vi "编辑控件.vi"(11 "控件类型":string) -> ()   [LabVIEW 2020]
panel:
  in  "图片路径":path
  in  "修改":bool
  in  "删除":bool
  in  "增加":bool
  in  "控件列表":i32(listbox)
  out "图片预览":picture
  in  "程序文本":string
  in  "关键字":string
  in  "控件名称":string
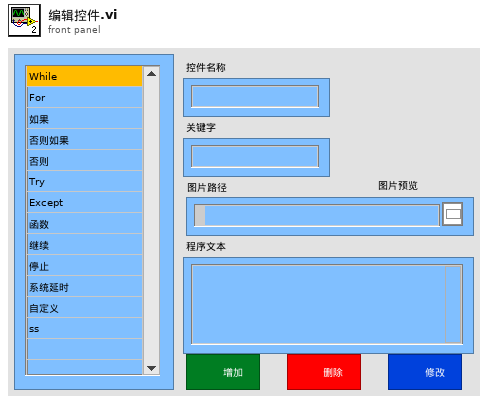
[diagram p1: front panel]
types:
  T1 = typedef "imagedata.ctl" = cluster{"image type":i32, "image depth":i32, "image":u8[], "mask":u8[], "colors":u32[], "Rectangle":cluster{"left":i16, "top":i16, "right":i16, "bottom":i16}}
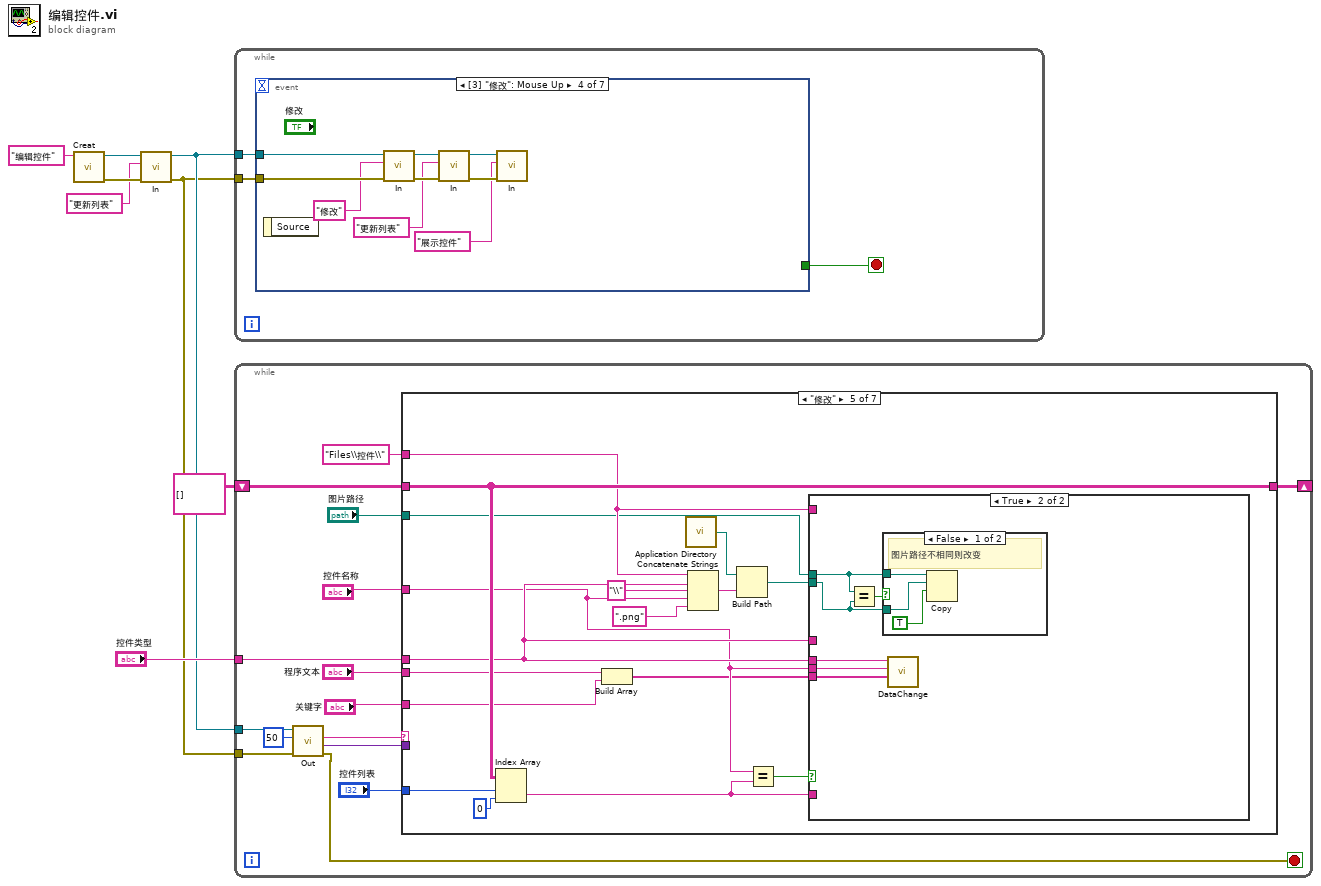
[diagram p0: block diagram]
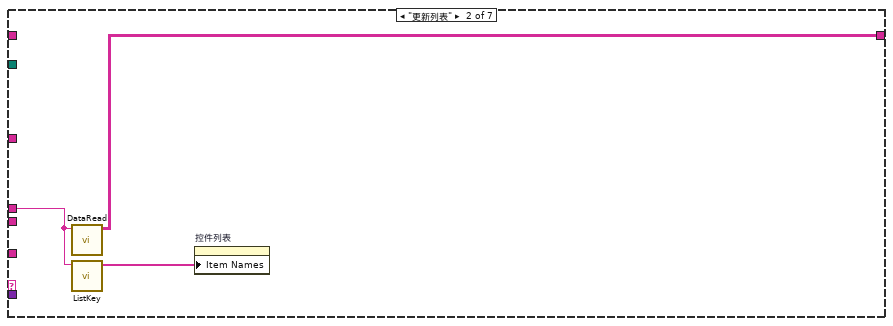
[diagram p3: hidden frame]
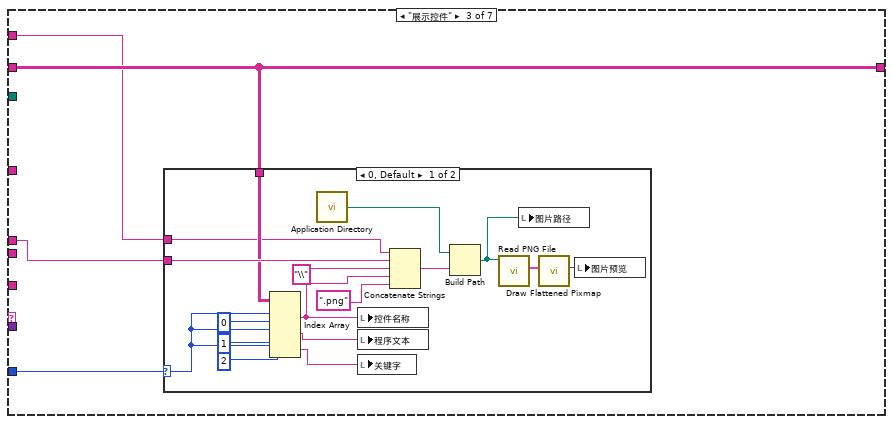
[diagram p4: hidden frame]
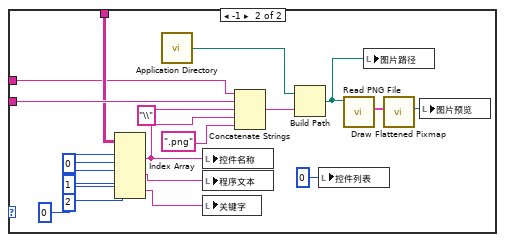
[diagram p5: hidden frame]
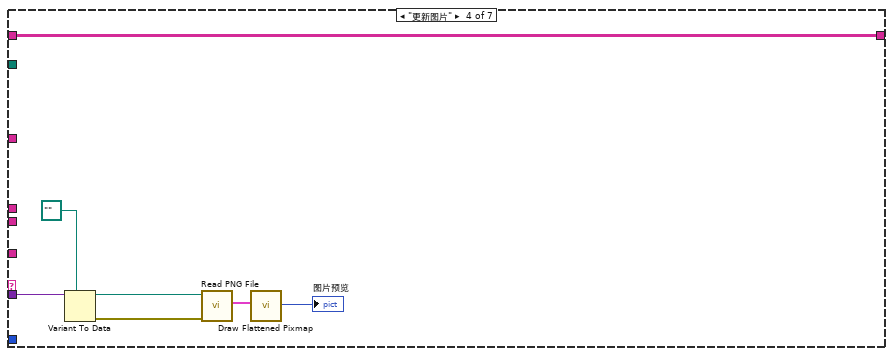
[diagram p6: hidden frame]
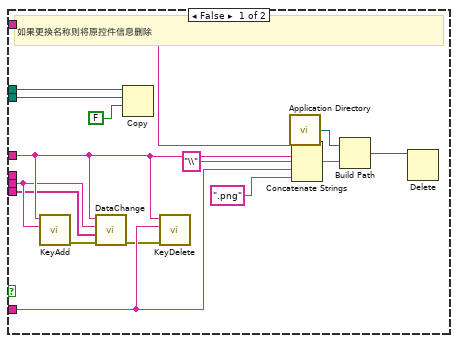
[diagram p7: hidden frame]
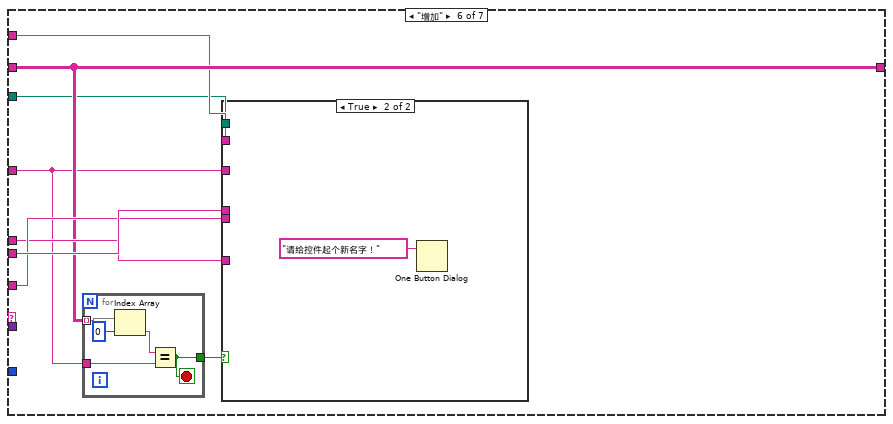
[diagram p9: hidden frame]
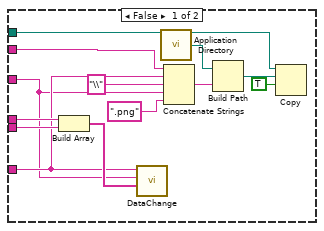
[diagram p10: hidden frame]
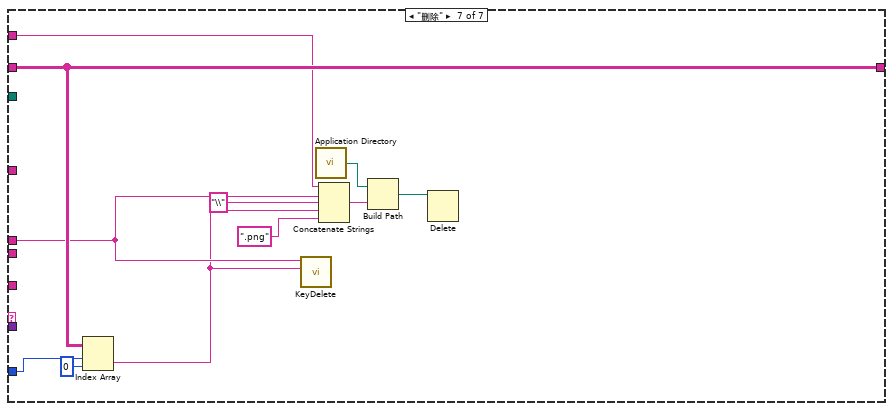
[diagram p11: hidden frame]
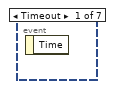
[diagram p12: hidden frame]
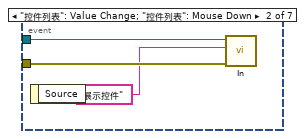
[diagram p13: hidden frame]
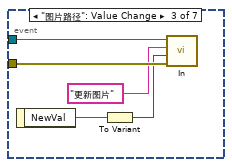
[diagram p14: hidden frame]
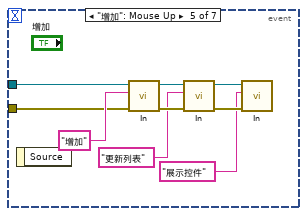
[diagram p15: hidden frame]
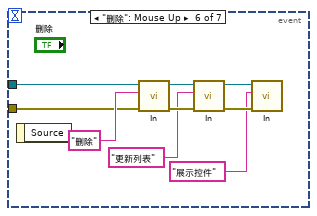
[diagram p16: hidden frame]
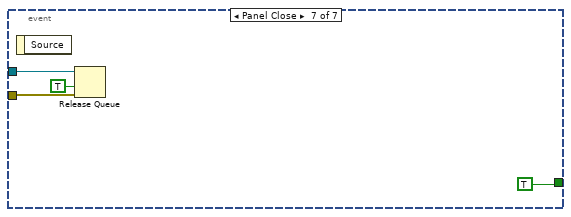
[diagram p17: hidden frame]
diagram:
  n1 = call "Creat.vi"("名称"="编辑控件") -> ("错误输出"=w2:errorcluster, "队列输出"=w5:refnum<queue>)  [unwired: 9 in]
  n2 = call "In.vi"("错误输入"=w2, "指令"="更新列表", "队列"=w5) -> ("错误输出"=w3:errorcluster, "队列输出"=w4:refnum<queue>)  [unwired: 7 in]
  n3 = while {
    tunnel: w4 -> [w11]
    tunnel: w3 -> [w10]
    stop <- w9 stop-if-true
    n4 = event shown="[3] \"修改\": Mouse Up" {
      selector: _ -> [_ _ _ _ _ _ _]
      dyn-events: _ -> [_ _ _ _ _ _ _]
      timeout: _ -> [_ _ _ _ _ _ _]
      tunnel: w11 -> [_ w14 w19 w28 w30 w39 w49]
      tunnel: w10 -> [_ w13 w18 w27 w29 w38 w48]
      tunnel: [_ _ _ _ _ _ TRUE] -> w9
      event Timeout {
        n5 = event-data() -> ()  [unwired: 1 in, 1 out]
      }
      event "控件列表": Value Change; "控件列表": Mouse Down {
        n6 = event-data() -> ()  [unwired: 1 in, 1 out]
        n7 = call "In.vi"("错误输入"=w13, "指令"="展示控件", "队列"=w14) -> ()  [unwired: 7 in, 2 out]
      }
      event "图片路径": Value Change {
        n8 = event-data() -> ("NewVal"=w17:path)  [unwired: 1 in]
        n9 = To Variant(anything=w17) -> (Variant=w15:variant)
        n10 = call "In.vi"("错误输入"=w18, "数据"=w15, "指令"="更新图片", "队列"=w19) -> ()  [unwired: 6 in, 2 out]
      }
      event "修改": Mouse Up {
        n11 = event-data() -> ()  [unwired: 1 in, 1 out]
        n12 = call "In.vi"("错误输入"=w27, "指令"="修改", "队列"=w28) -> ("错误输出"=w24:errorcluster, "队列输出"=w25:refnum<queue>)  [unwired: 7 in]
        n13 = call "In.vi"("错误输入"=w24, "指令"="更新列表", "队列"=w25) -> ("错误输出"=w22:errorcluster, "队列输出"=w23:refnum<queue>)  [unwired: 7 in]
        n14 = call "In.vi"("错误输入"=w22, "指令"="展示控件", "队列"=w23) -> ()  [unwired: 7 in, 2 out]
      }
      event "增加": Mouse Up {
        n15 = event-data() -> ()  [unwired: 1 in, 1 out]
        n16 = call "In.vi"("错误输入"=w29, "指令"="增加", "队列"=w30) -> ("错误输出"=w35:errorcluster, "队列输出"=w36:refnum<queue>)  [unwired: 7 in]
        n17 = call "In.vi"("错误输入"=w35, "指令"="更新列表", "队列"=w36) -> ("错误输出"=w33:errorcluster, "队列输出"=w34:refnum<queue>)  [unwired: 7 in]
        n18 = call "In.vi"("错误输入"=w33, "指令"="展示控件", "队列"=w34) -> ()  [unwired: 7 in, 2 out]
      }
      event "删除": Mouse Up {
        n19 = event-data() -> ()  [unwired: 1 in, 1 out]
        n20 = call "In.vi"("错误输入"=w38, "指令"="删除", "队列"=w39) -> ("错误输出"=w44:errorcluster, "队列输出"=w45:refnum<queue>)  [unwired: 7 in]
        n21 = call "In.vi"("错误输入"=w44, "指令"="更新列表", "队列"=w45) -> ("错误输出"=w42:errorcluster, "队列输出"=w43:refnum<queue>)  [unwired: 7 in]
        n22 = call "In.vi"("错误输入"=w42, "指令"="展示控件", "队列"=w43) -> ()  [unwired: 7 in, 2 out]
      }
      event Panel Close {
        n23 = event-data() -> ()  [unwired: 1 in, 1 out]
        n24 = Release Queue(queue=w49, force destroy? (F)=TRUE ("强制销毁？(F)"), error in (no error)=w48) -> ()  [unwired: 3 out]
      }
    }
  }
  n25 = while {
    tunnel: w4 -> [w58]
    tunnel: w3 -> [w57]
    shift-right: [w65] -> _
    shift-left: string[][] [] ("数据") -> [w64]
    tunnel: "控件类型" -> [w63]
    stop <- w54 stop-if-true
    n26 = call "Out.vi"("错误输入"=w57, "超时毫秒(-1)"=50, "队列"=w58) -> ("错误输出"=w54:errorcluster, "数据"=w55:variant, "指令"=w56:string)  [unwired: 5 in, 1 out]
    n27 = case shown="\"修改\"" w56 {
      tunnel: w55 -> [_ _ _ w110 _ _ _]
      tunnel: [w66 w68 w72 w114 w128 w161 w194] -> w65
      tunnel: w64 -> [w66 _ w72 w114 w128 w161 w194]
      tunnel: w63 -> [_ w69 w73 _ w118 w162 w187]
      tunnel: "控件名称" -> [_ _ _ _ w117 w160 _]
      tunnel: "程序文本" -> [_ _ _ _ w126 w164 _]
      tunnel: "关键字" -> [_ _ _ _ w125 w163 _]
      tunnel: "控件列表" -> [_ _ w71 _ w124 _ w193]
      tunnel: "Files\\控件\\" ("名称或相对路径") -> [_ _ w70 _ w121 w158 w184]
      tunnel: "图片路径" -> [_ _ _ _ w119 w157 _]
      frame "null", Default {
      }
      frame "更新列表" {
        n28 = call "DataRead.vi"("段名"=w69) -> ("数据"=w68:string[][])  [unwired: 10 in]
        n29 = call "ListKey.vi"("section"=w69) -> ("keys"=w67:string[])  [unwired: 10 in]
        n30 = property on="控件列表" class="LstBox (strict)"("Item Names"=w67) -> ()  [unwired: 2 in, 2 out]
      }
      frame "展示控件" {
        n31 = case shown="0, Default" w71 {
          selector: w71 -> [w75 _]
          tunnel: w73 -> [w78 w96]
          tunnel: w72 -> [w76 w94]
          tunnel: w70 -> [w74 w91]
          frame 0, Default {
            n32 = Index Array(array=w76, index (row) #1=w75, index (col) #1=0 ("禁用的索引 (列)"), index (row) #2=w75, index (col) #2=1 ("禁用的索引 (列)"), index (row) #3=w75, index (col) #3=2 ("禁用的索引 (列)")) -> (element #1=w77:string, element #2=w89:string, element #3=w90:string)
            n33 = call <vilib>:"Application Directory.vi"() -> ("Application Directory"=w79:path)
            n34 = local write "控件名称"(w77) -> ()
            n35 = local write "程序文本"(w89) -> ()
            n36 = local write "关键字"(w90) -> ()
            n37 = Concatenate Strings(w74, w78, "\\" ("字符串"), w77, ".png" ("字符串")) -> (w80:string)
            n38 = Build Path(base path=w79, name or relative path=w80) -> (appended path=w85:path)
            n39 = call <vilib>:"Read PNG File.vi"("path to PNG file"=w85) -> ("image data"=w83:T1)  [unwired: 8 in, 2 out]
            n40 = local write "图片路径"(w85) -> ()
            n41 = call <vilib>:"Draw Flattened Pixmap.vi"("image data"=w83) -> ("new picture"=w84:picture)  [unwired: 8 in]
            n42 = local write "图片预览"(w84) -> ()
          }
          frame -1 {
            w93 = 0 ("禁用的索引 (列)")
            n43 = Index Array(array=w94, index (row) #1=w93, index (col) #1=0 ("禁用的索引 (列)"), index (row) #2=w93, index (col) #2=1 ("禁用的索引 (列)"), index (row) #3=w93, index (col) #3=2 ("禁用的索引 (列)")) -> (element #1=w95:string, element #2=w107:string, element #3=w108:string)
            n44 = call <vilib>:"Application Directory.vi"() -> ("Application Directory"=w97:path)
            n45 = local write "控件名称"(w95) -> ()
            n46 = local write "程序文本"(w107) -> ()
            n47 = local write "关键字"(w108) -> ()
            n48 = Concatenate Strings(w91, w96, "\\" ("字符串"), w95, ".png" ("字符串")) -> (w98:string)
            n49 = Build Path(base path=w97, name or relative path=w98) -> (appended path=w103:path)
            n50 = local write "控件列表"(0 ("控件列表")) -> ()
            n51 = call <vilib>:"Read PNG File.vi"("path to PNG file"=w103) -> ("image data"=w101:T1)  [unwired: 8 in, 2 out]
            n52 = local write "图片路径"(w103) -> ()
            n53 = call <vilib>:"Draw Flattened Pixmap.vi"("image data"=w101) -> ("new picture"=w102:picture)  [unwired: 8 in]
            n54 = local write "图片预览"(w102) -> ()
          }
        }
      }
      frame "更新图片" {
        n55 = Variant To Data(type=path "" ("类型"), Variant=w110) -> (data=w113:path, error out=w109:errorcluster)  [unwired: 1 in]
        n56 = call <vilib>:"Read PNG File.vi"("error in (no error)"=w109, "path to PNG file"=w113) -> ("image data"=w115:T1)  [unwired: 7 in, 2 out]
        n57 = call <vilib>:"Draw Flattened Pixmap.vi"("image data"=w115) -> ("new picture"=→"图片预览":picture)  [unwired: 8 in]
      }
      frame "修改" {
        n58 = Index Array(array=w128, index (row)=w124, index (col)=0 ("禁用的索引 (列)")) -> (element=w122:string)
        n59 = Build Array(w126, w125) -> (w116:string[])
        n60 = call <vilib>:"Application Directory.vi"() -> ("Application Directory"=w131:path)
        n61 = Concatenate Strings(w121, w118, "\\" ("字符串"), w117, ".png" ("字符串")) -> (w132:string)
        n62 = Build Path(base path=w131, name or relative path=w132) -> (appended path=w120:path)
        n63 = Equal?(x=w117, y=w122) -> (x = y?=w123:bool)
        n64 = case shown="True" w123 {
          tunnel: w118 -> [w137 _]
          tunnel: w122 -> [w142 _]
          tunnel: w121 -> [w141 _]
          tunnel: w120 -> [w139 w148]
          tunnel: w119 -> [w138 w149]
          tunnel: w118 -> [_ w153]
          tunnel: w117 -> [w136 w152]
          tunnel: w116 -> [w135 w151]
          frame False {
            # "如果更换名称则将原控件信息删除"
            n65 = call "KeyAdd.vi"("键名"=w136, "段名"=w137) -> ("error out"=w134:errorcluster)  [unwired: 9 in]
            n66 = call "DataChange.vi"("error in (no error)"=w134, "值"=w135, "键名"=w136, "段名"=w137) -> ("error out"=w133:errorcluster)  [unwired: 7 in]
            n67 = Copy(9:FALSE ("覆盖(F)"), 10:w139, 11:w138) -> ()  [unwired: 2 in, 3 out]
            n68 = call "KeyDelete.vi"("error in (no error)"=w133, "键名"=w142, "段名"=w137) -> ()  [unwired: 8 in, 1 out]
            n69 = call <vilib>:"Application Directory.vi"() -> ("Application Directory"=w145:path)
            n70 = Concatenate Strings(w141, w137, "\\" ("字符串"), w142, ".png" ("字符串")) -> (w144:string)
            n71 = Build Path(base path=w145, name or relative path=w144) -> (appended path=w143:path)
            n72 = Delete(path (use dialog)=w143) -> ()  [unwired: 4 in, 3 out]
          }
          frame True {
            n73 = Equal?(x=w149, y=w148) -> (x = y?=w150:bool)
            n74 = case shown="False" w150 {
              tunnel: w149 -> [w156 _]
              tunnel: w148 -> [w155 _]
              frame False {
                # "图片路径不相同则改变"
                n75 = Copy(9:TRUE ("覆盖(F)"), 10:w155, 11:w156) -> ()  [unwired: 2 in, 3 out]
              }
              frame True {
                # "图片路径相同则不改"
              }
            }
            n76 = call "DataChange.vi"("值"=w151, "键名"=w152, "段名"=w153) -> ()  [unwired: 8 in, 1 out]
          }
        }
      }
      frame "增加" {
        n77 = for {
          tunnel: w161 -> [w169] mode=indexing
          tunnel: w160 -> [w166]
          tunnel: [w165] -> w159
          stop <- w165 stop-if-true
          n78 = Index Array(array=w169, index=0 ("索引")) -> (element=w167:string)
          n79 = Equal?(x=w167, y=w166) -> (x = y?=w165:bool)
        }
        n80 = case shown="True" w159 {
          tunnel: w164 -> [w182 _]
          tunnel: w163 -> [w181 _]
          tunnel: w162 -> [w175 _]
          tunnel: w160 -> [w171 _]
          tunnel: w157 -> [w173 _]
          tunnel: w158 -> [w170 _]
          frame False {
            n81 = Build Array(w182, w181) -> (w180:string[])
            n82 = call "DataChange.vi"("值"=w180, "键名"=w171, "段名"=w175) -> ()  [unwired: 8 in, 1 out]
            n83 = call <vilib>:"Application Directory.vi"() -> ("Application Directory"=w178:path)
            n84 = Concatenate Strings(w170, w175, "\\" ("字符串"), w171, ".png" ("字符串")) -> (w179:string)
            n85 = Build Path(base path=w178, name or relative path=w179) -> (appended path=w174:path)
            n86 = Copy(9:TRUE ("覆盖(F)"), 10:w174, 11:w173) -> ()  [unwired: 2 in, 3 out]
          }
          frame True {
            n87 = One Button Dialog(message="请给控件起个新名字！" ("消息")) -> ()  [unwired: 1 in, 1 out]
          }
        }
      }
      frame "删除" {
        n88 = Index Array(array=w194, index (row)=w193, index (col)=0 ("禁用的索引 (列)")) -> (element=w185:string)
        n89 = call "KeyDelete.vi"("键名"=w185, "段名"=w187) -> ()  [unwired: 9 in, 1 out]
        n90 = call <vilib>:"Application Directory.vi"() -> ("Application Directory"=w190:path)
        n91 = Concatenate Strings(w184, w187, "\\" ("字符串"), w185, ".png" ("字符串")) -> (w191:string)
        n92 = Build Path(base path=w190, name or relative path=w191) -> (appended path=w186:path)
        n93 = Delete(path (use dialog)=w186) -> ()  [unwired: 4 in, 3 out]
      }
    }
  }
